vi "Check Finish Game.vi"(7 "Game Result":refnum<vi>, 8 "error in (no error)":errorcluster, 11 "Application in":refnum<class "Application.lvclass">) -> (0 "error out":errorcluster, 2 "Finish Game?":bool, 3 "Application out":refnum<class "Application.lvclass">)   [LabVIEW 2021, in "Application.lvclass"]
uses:
  Application.lvclass
  Application.lvclass/Application.ctl
  Board Game_class/Board Game.lvclass
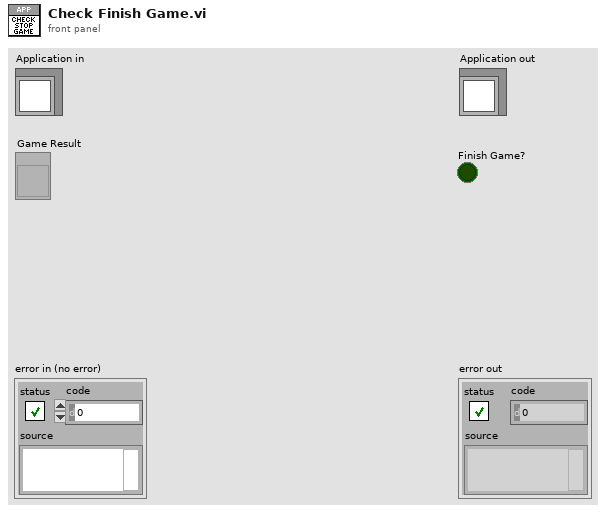
[diagram p1: front panel]
types:
  T1 = typedef "Application.lvclass/Packed Refs.ctl" = cluster{"graphics queue":refnum<queue>, "Pause Game Event":refnum<user-event>, "Stop Control Loop":refnum<user-event>, "Direction":refnum<notifier>, "play sound":refnum<user-event>, "stop sound":refnum<user-event>, "Timer":refnum<data-value>}
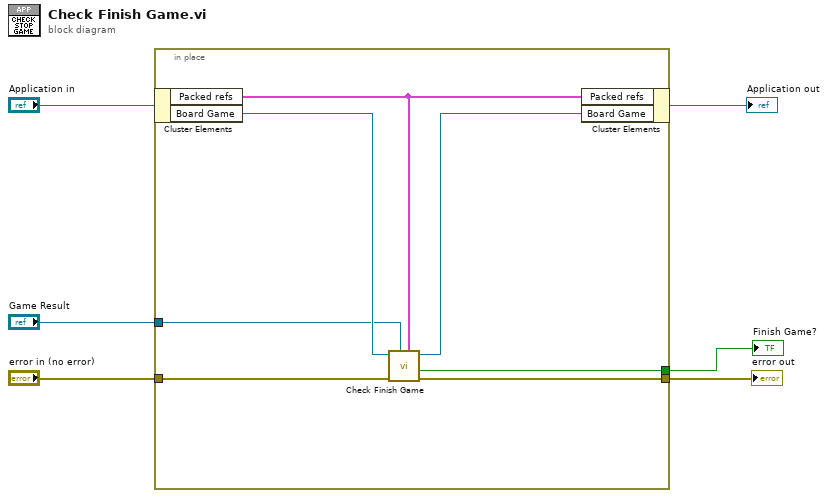
[diagram p0: block diagram]
diagram:
  n1 = in-place {
    in-place-border: "error in (no error)" -> [w11]
    in-place-border: [w10] -> w4
    in-place-border: [w8] -> w2
    in-place-border: "Game Result" -> [w7]
    n2 = in-place-cluster #1("Application in") -> ("Packed refs"=w9:T1, "Board Game"=w13:refnum<class "Board Game.lvclass">)
    n3 = call "Check Finish Game.vi"("Packed refs"=w9, "Game Result"=w7, "error in (no error)"=w11, "Board Game in"=w13) -> ("error out"=w10:errorcluster, "Finish Game?"=w8:bool, "Board Game out"=w12:refnum<class "Board Game.lvclass">)  [unwired: 5 in]
    n4 = in-place-cluster #1("Packed refs"=w9, "Board Game"=w12) -> (→"Application out":refnum<class "Application.lvclass">)
  }
  "error out" <- w4
  "Finish Game?" <- w2
